vi "skalowanie czasu enkoderow.vi"(7 "mnoznik (1)":dbl=1.0 format="%#_13g", 11 "data":waveform(dbl)[](array[waveform])) -> (2 "t0":timestamp, 3 "dT out":dbl)   [LabVIEW 2014]
doc: "Skaluje czas dT enkoderów\nna podstawie rzeczywistych wartoœci dT przebiegów analogowych"
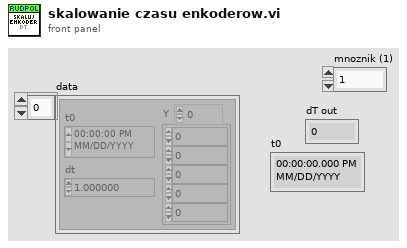
[diagram p1: front panel]
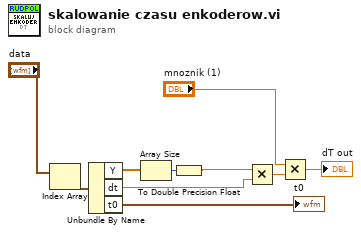
[diagram p0: block diagram]
diagram:
  n1 = Index Array(array="data") -> (element=w6:waveform(dbl))  [unwired: 1 in]
  n2 = Unbundle By Name(w6) -> ("Y"=w9:dbl[], "dt"=w10:dbl, "t0"=→"t0":timestamp)
  n3 = Array Size(array=w9) -> (size(s)=w5:i32)
  n4 = To Double Precision Float(number=w5) -> (double precision float=w1:dbl)
  n5 = Multiply(x=w1, y=w10) -> (x*y=w4:dbl)
  n6 = Multiply(x="mnoznik (1)", y=w4) -> (x*y=→"dT out":dbl)
